vi "Remove duplicate comments in sxp file.vi"() -> ()   [LabVIEW 2020]
panel:
  in  "path":path
  out "file path out":path
  out "error out":errorcluster
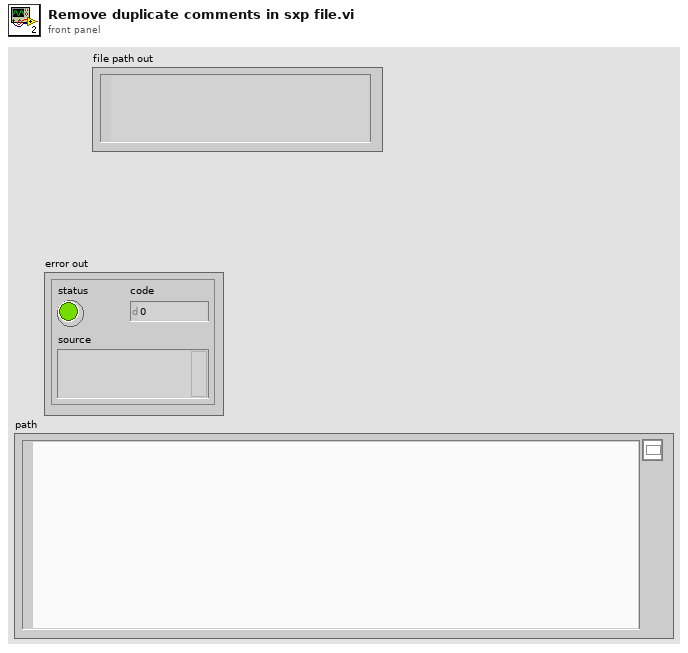
[diagram p1: front panel]
types:
  T1 = enum16{"open", "replace", "create", "open or create", "replace or create", "replace or create with confirmation"}
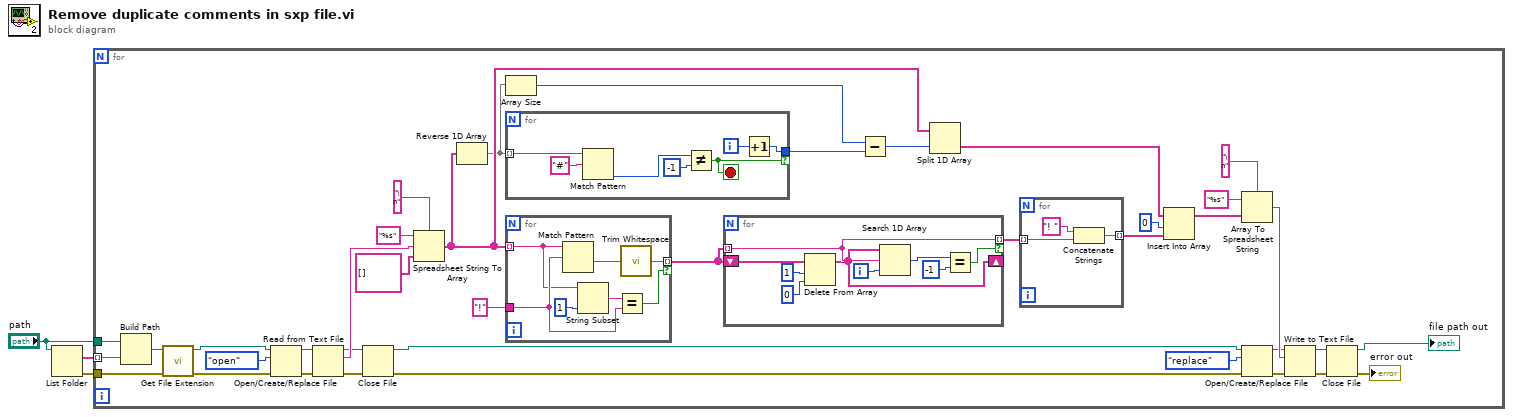
[diagram p0: block diagram]
diagram:
  n1 = List Folder(path="path") -> (filenames=w3:string[], error out=w2:errorcluster)  [unwired: 3 in, 2 out]
  n2 = for {
    tunnel: w3 -> [w16] mode=indexing
    tunnel: w2 -> [w15]
    tunnel: "path" -> [w14]
    n3 = Build Path(base path=w14, name or relative path=w16) -> (appended path=w19:path)
    n4 = call <vilib>:"Get File Extension.vi"("error in (no error)"=w15, "file"=w19) -> ("error out"=w18:errorcluster, "dup file"=w17:path)  [unwired: 5 in, 3 out]
    n5 = Open/Create/Replace File(file path (use dialog)=w17, error in=w18, operation (0:open)=T1."open") -> (refnum out=w37:refnum<file>, error out=w36:errorcluster)  [unwired: 3 in, 1 out]
    n6 = Read from Text File(file (use dialog)=w37, error in=w36) -> (refnum out=w25:refnum<file>, text=w35:string, error out=w26:errorcluster)  [unwired: 2 in, 1 out]
    n7 = Close File(refnum=w25, error in=w26) -> (path=w24:path, error out=w23:errorcluster)
    n8 = Spreadsheet String To Array(delimiter (Tab)="\n", format string="%s", spreadsheet string=w35, array type (2D Dbl)=string[] []) -> (array=w11:string[])
    n9 = Reverse 1D Array(array=w11) -> (reversed array=w6:string[])
    n10 = Array Size(array=w6) -> (size(s)=w7:i32)
    n11 = for {
      tunnel: w6 -> [w52] mode=indexing
      tunnel: [w46] -> w8 if=w48
      i -> [w47]
      stop <- w48 stop-if-true
      n12 = Match Pattern(string=w52, regular expression="#") -> (offset past match=w50:i32)  [unwired: 1 in, 3 out]
      n13 = Not Equal?(x=w50, y=-1) -> (x != y?=w48:bool)
      n14 = Increment(x=w47) -> (x+1=w46:i32)
    }
    n15 = for {
      tunnel: w11 -> [w64] mode=indexing
      tunnel: [w62] -> w13 mode=indexing if=w66
      tunnel: "!" ("Comment character 2") -> [w65]
      n16 = Match Pattern(string=w64, regular expression=w65) -> (after substring=w63:string)  [unwired: 1 in, 3 out]
      n17 = String Subset(string=w64, length (rest)=1 ("length (rest)")) -> (substring=w67:string)  [unwired: 1 in]
      n18 = Equal?(x=w67, y=w65) -> (x = y?=w66:bool)
      n19 = call <vilib>:"Trim Whitespace.vi"("string"=w63) -> ("trimmed string"=w62:string)  [unwired: 1 in]
    }
    n20 = for {
      tunnel: w13 -> [w57] mode=indexing
      tunnel: [w57] -> w5 mode=indexing if=w56
      shift-right: [w55] -> _
      shift-left: w13 -> [w59]
      i -> [w54]
      n21 = Delete From Array(array=w59, length=1, index=0) -> (array with subset deleted=w55:string[])  [unwired: 1 out]
      n22 = Search 1D Array(1D array=w55, element=w57, start index (0)=w54) -> (index of element=w60:i32)
      n23 = Equal?(x=w60, y=-1) -> (x = y?=w56:bool)
    }
    n24 = Subtract(x=w7, y=w8) -> (x-y=w12:i32)
    n25 = Split 1D Array(array=w11, index=w12) -> (second subarray=w10:string[])  [unwired: 1 out]
    n26 = for {
      tunnel: w5 -> [w45] mode=indexing
      tunnel: [w43] -> w4 mode=indexing
      n27 = Concatenate Strings("! " ("string"), w45) -> (w43:string)
    }
    n28 = Insert Into Array(array=w10, index=0, new element=w4) -> (w29:string[])
    n29 = Array To Spreadsheet String(delimiter (Tab)="\n", array=w29, 3:"%s" ("format string")) -> (spreadsheet string=w31:string)
    n30 = Open/Create/Replace File(file path (use dialog)=w24, error in=w23, operation (0:open)=T1."replace") -> (refnum out=w22:refnum<file>, error out=w21:errorcluster)  [unwired: 3 in, 1 out]
    n31 = Write to Text File(file (use dialog)=w22, text=w31, error in=w21) -> (refnum out=w34:refnum<file>, error out=w33:errorcluster)  [unwired: 1 in, 1 out]
    n32 = Close File(refnum=w34, error in=w33) -> (path=→"file path out":path, error out=→"error out":errorcluster)
  }
